vi "test Get Set RAF CD.vi"(8 "error in (no error)":errorcluster, 11 "TestCase in":refnum<class "Switch Scripting Test Case.lvclass">) -> (0 "error out":errorcluster, 3 "TestCase out":refnum<class "Switch Scripting Test Case.lvclass">)   [LabVIEW 2017, in "Switch Scripting Test Case.lvclass"]
uses:
  Switch Scripting Test Case.lvclass
  Shared/Routing and Faulting Custom Device Settings.ctl
  Switch Scripting Test Case.lvclass/Switch Scripting Test Case.ctl
  <vilib>/addons/_JKI Toolkits/VI Tester/TestCase.llb/TestCase.lvclass
  Scripting/Scripting/Switch Scripting.lvlib
  Shared/Switch Shared.lvlib
  C:/Program Files (x86)/National Instruments/LabVIEW 2017/vi.lib/addons/_JKI Toolkits/VI Tester/TestCase.llb/TestCase.lvclass
panel:
  in  "Save?":bool
  out "Output Filename":string
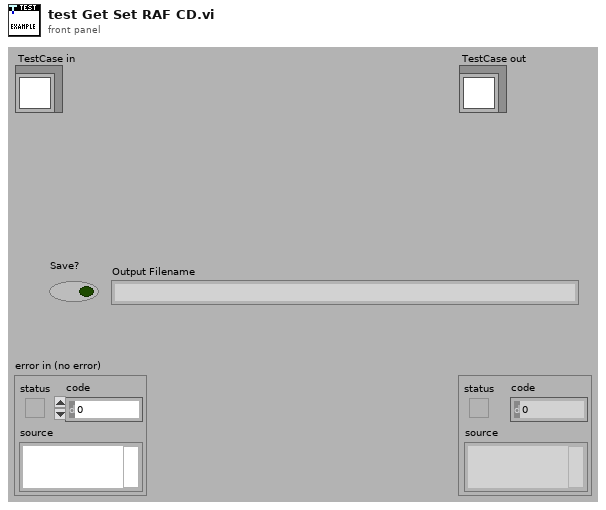
[diagram p1: front panel]
types:
  T1 = typedef "Switch Shared.lvlib/Routing and Faulting Custom Device Settings.ctl" = cluster{"Name":string}
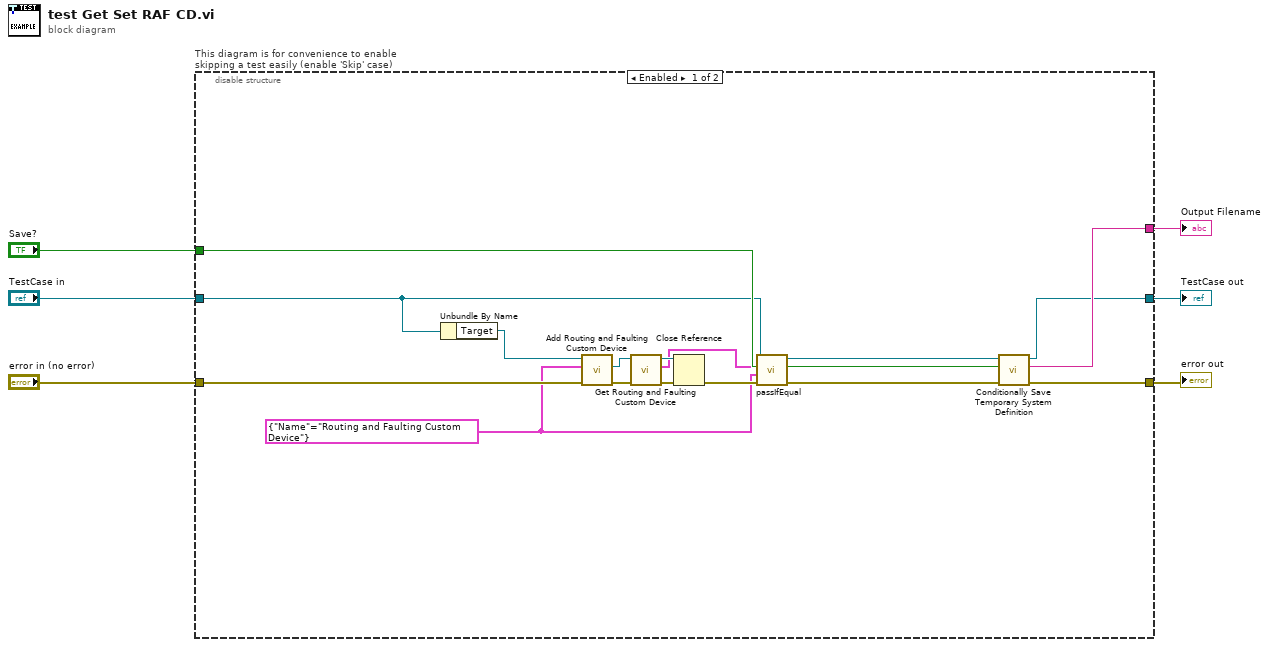
[diagram p0: block diagram]
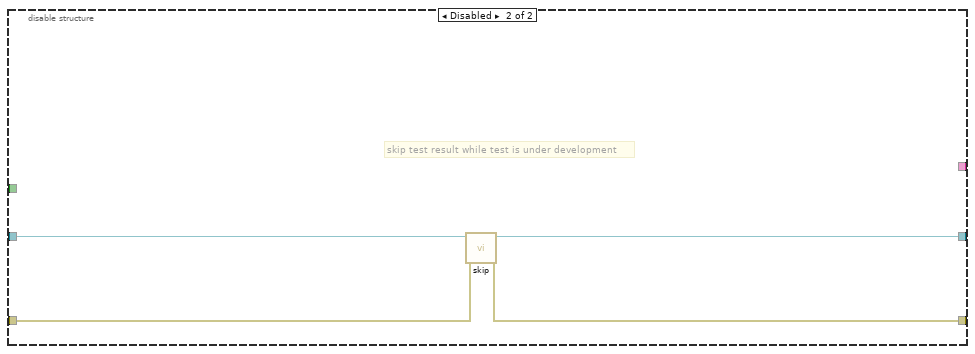
[diagram p2: hidden frame]
diagram:
  n1 = disable-structure "This diagram is for convenience to enable skipping a test easily (enable 'Skip' case)" shown="Enabled" {
    disable-tunnel: "TestCase in" -> [w13 w26]
    disable-tunnel: [w11 w24] -> w3
    disable-tunnel: [w21 w25] -> w5
    disable-tunnel: "error in (no error)" -> [w22 w23]
    disable-tunnel: [w20 _] -> w2
    disable-tunnel: "Save?" -> [w19 _]
    frame Enabled {
      w7 = T1 {"Name"="Routing and Faulting Custom Device"} ("Routing and Faulting Custom Device Settings")
      n2 = Unbundle By Name(w13) -> ("Target"=w12:refnum<k24>)
      n3 = call "Add Routing and Faulting Custom Device.vi"("error in (no error)"=w22, "Settings"=w7, "Target in"=w12) -> ("error out"=w17:errorcluster, "RAF Custom Device"=w16:refnum<k24>)  [unwired: 6 in, 1 out]
      n4 = call "Get Routing and Faulting Custom Device.vi"("error in (no error)"=w17, "RAF Custom Device in"=w16) -> ("error out"=w9:errorcluster, "Settings"=w15:T1, "RAF Custom Device out"=w18:refnum<k24>)  [unwired: 7 in]
      n5 = Close Reference(reference=w18, error in (no error)=w9) -> (error out=w8:errorcluster)
      n6 = call-dynamic "passIfEqual.vi"("error in (no error)"=w8, "y"=w7, "x"=w15, "TestCase in"=w13) -> ("error out"=w10:errorcluster, "TestCase out"=w14:refnum<class "Switch Scripting Test Case.lvclass">)  [unwired: 6 in]
      n7 = call "Conditionally Save Temporary System Definition.vi"("error in (no error)"=w10, "Save?"=w19, "Test Case"=w14) -> ("error out"=w21:errorcluster, "filename"=w20:string, "Test Case"=w11:refnum<class "Switch Scripting Test Case.lvclass">)  [unwired: 6 in]
    }
    frame Disabled {
      # "skip test result while test is under development"
      n8 = call <vilib>:"skip.vi"("error in (no error)"=w23, "TestCase in"=w26) -> ("error out"=w25:errorcluster, "TestCase out"=w24:refnum<class "Switch Scripting Test Case.lvclass">)  [unwired: 8 in]
    }
  }
  "error out" <- w5
  "TestCase out" <- w3
  "Output Filename" <- w2
